vi "CRYAPI MSG PRO.vi"() -> ()   [LabVIEW 2013]
uses:
  CRYMain Sub Window Global.vi
  CRYProject/CRYProject Editor Global.vi
  CRYStepSetup/CRYStepSetup Global.vi
panel:
  in  "bStepRecovery":bool=TRUE
  in  "bOpenProjectFullPath":bool=TRUE
  in  "bStop":bool=TRUE
  in  "bMsg":bool=TRUE
  in  "nDData":i32
  in  "nSData":i32
  in  "sData":string="REMOTE_COMMAND"
  in  "nData":i32
  in  "pVI":refnum<vi>
  in  "sMsgCommand":string="REMOTE_COMMAND"
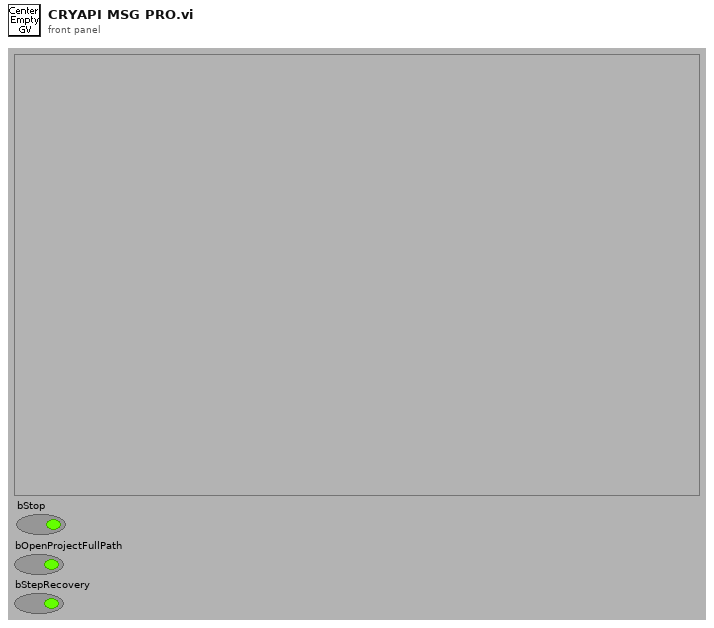
[diagram p1: front panel]
types:
  T1 = enum32{"Invalid", "Standard", "Closed", "Hidden", "Minimized", "Maximized"}
  T2 = typedef "LVRectTypeDef.ctl" = cluster{"Left":i16, "Top":i16, "Right":i16, "Bottom":i16}
  T3 = cluster{"nType":i32, "nParent":i32, "pVIW":refnum<vi>, "pSPW":refnum<vi>, "nTypeF":i32, "pVIF":refnum<vi>, "pSPF":refnum<vi>, "nIDSpliter":i32, "nProperty":i32, "Bound":T2, "nID":i32, "nData":i32, "sData":string, "pWVI":refnum<vi>, "sTitle":string, "cPages":cluster{"nPage":i32, "sTitle":string, "sIcon":string, "pVI":refnum<vi>, "nID":i32}[], "pTab":refnum<vi>, "nIDPages":i32[], "pSPT":refnum<vi>, "sTemp":string, "nDockID":i32, "nDockLR":i32, "sIcon":string}
  T4 = cluster{"EventName":string, "Arg1":string, "Numeric":u16, "Numeric 2":u16, "AddSteps ":refnum<vi>, "Arg1 2":string, "Arg1 3":string, "Boolean":bool}
  T5 = cluster{"sStepName":string, "nStepVINo":i32, "nStepVINoDisplay":i32}
  T6 = typedef "CRYTS.ctl" = cluster{"No.TS":u16, "TS File Path":path, "TS Name":string, "EditStepName":string, "Steps":T7[], "New State":bool, "Change State":bool, "Flattened CurveLib Data":string, "Document Data":string, "EditStepNo":u16, "Operator Start File":string, "Sequence Type":string, "Sequence Language":string}
  T7 = typedef "CRYStep.ctl" = cluster{"No.VI":i32, "Category":string, "StepName":string, "Seq setup flattened":string, "Comment":string, "Steps config.":bool[], "Jump config":i32[], "Start":dbl, "Increment":dbl, "Name":string, "Unit":string, "Y data":u16, "Y prefix":string, "Y dB ref":dbl, "Y unit":string, "Repeat State Array":cluster{"Start":dbl, "Increment":dbl, "Count":i32, "Num":i32}[]}
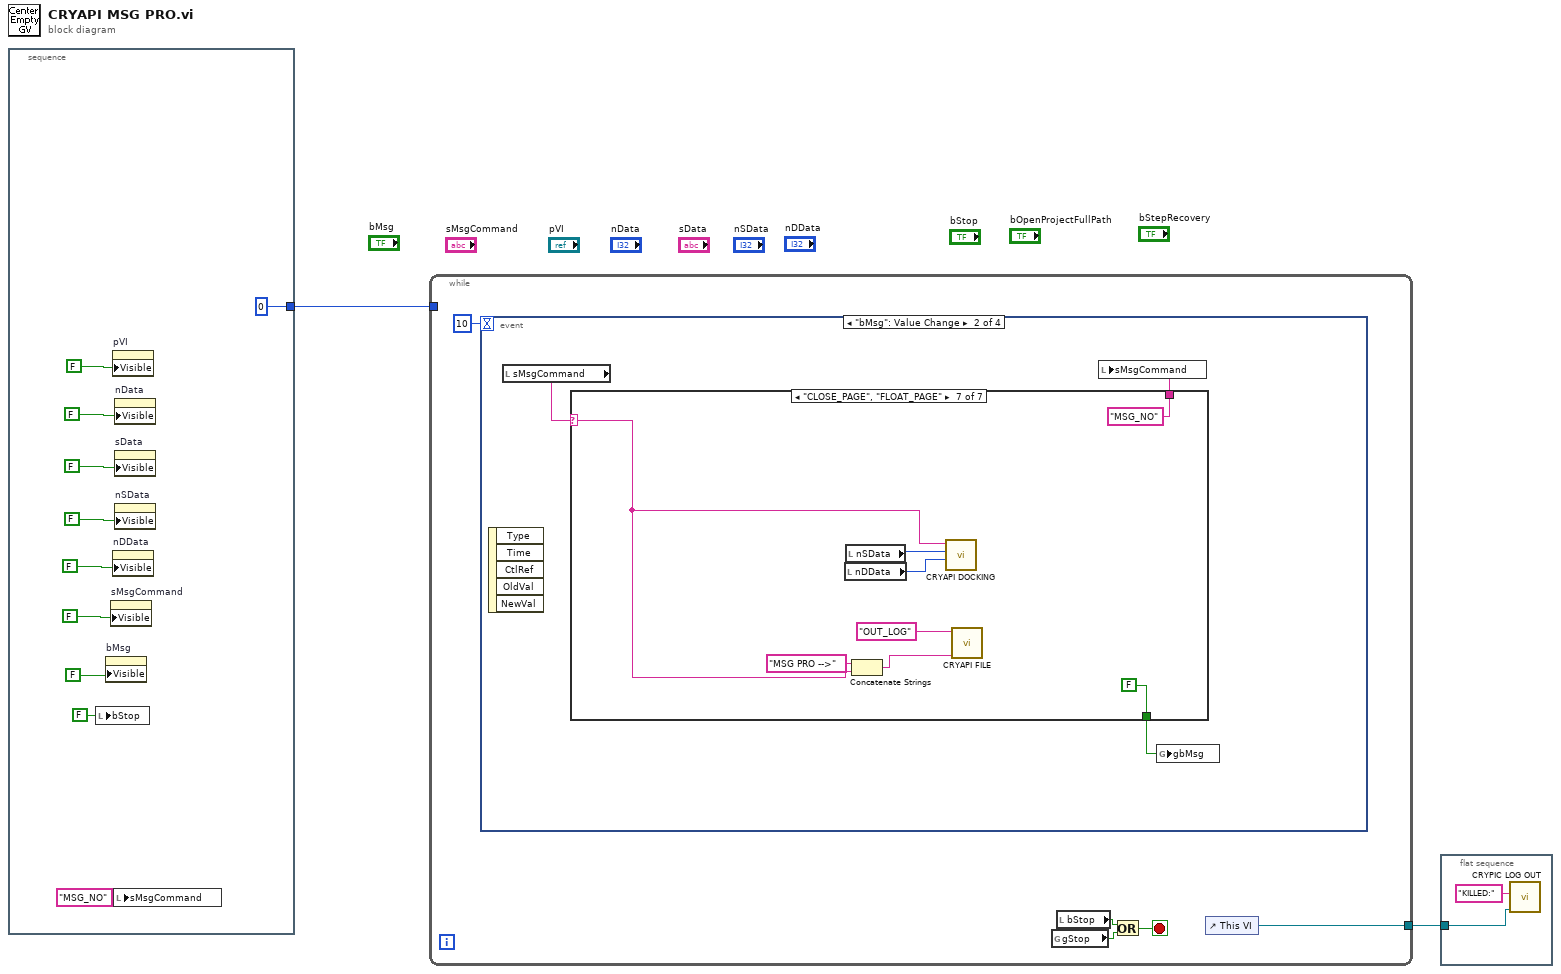
[diagram p0: block diagram]
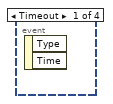
[diagram p2: hidden frame]
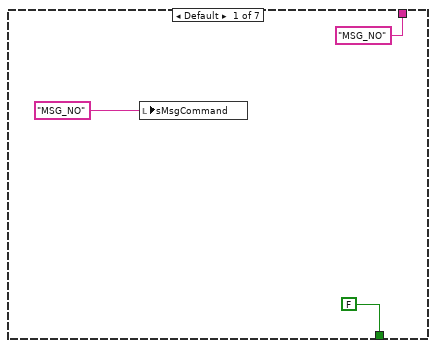
[diagram p3: hidden frame]
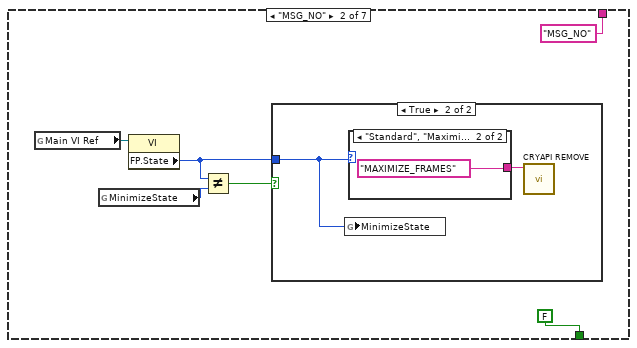
[diagram p4: hidden frame]
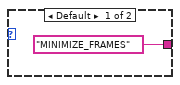
[diagram p6: hidden frame]
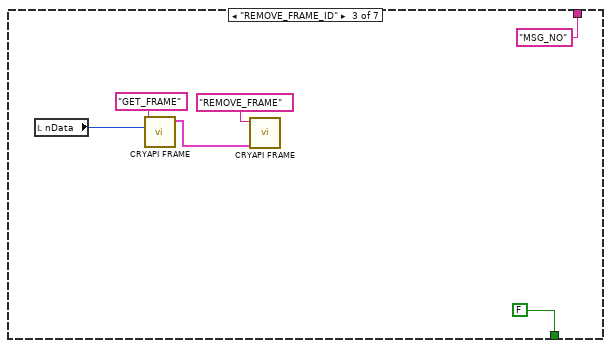
[diagram p7: hidden frame]
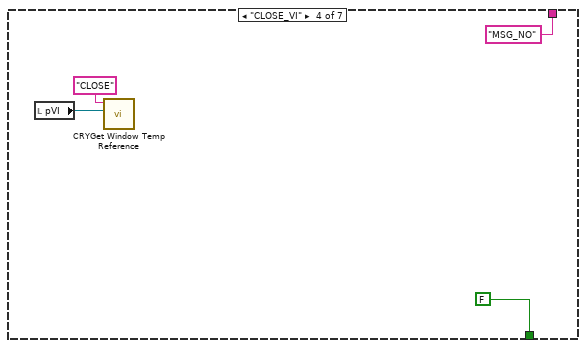
[diagram p8: hidden frame]
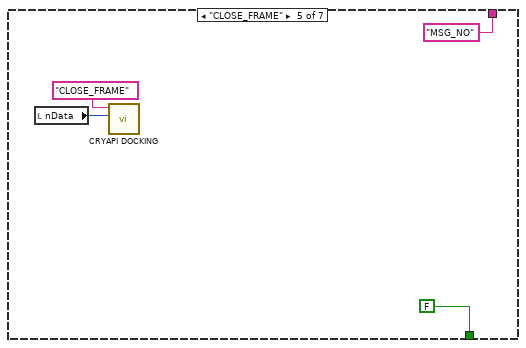
[diagram p9: hidden frame]
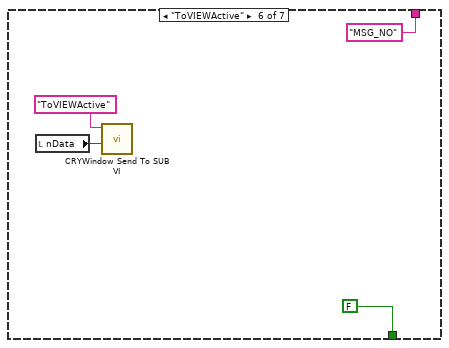
[diagram p10: hidden frame]
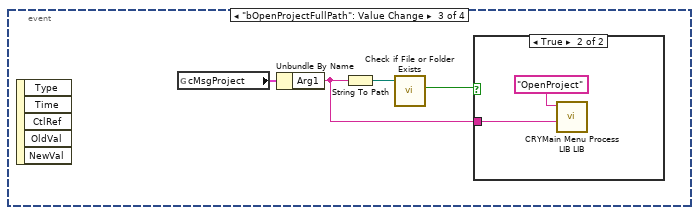
[diagram p11: hidden frame]
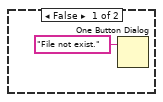
[diagram p12: hidden frame]
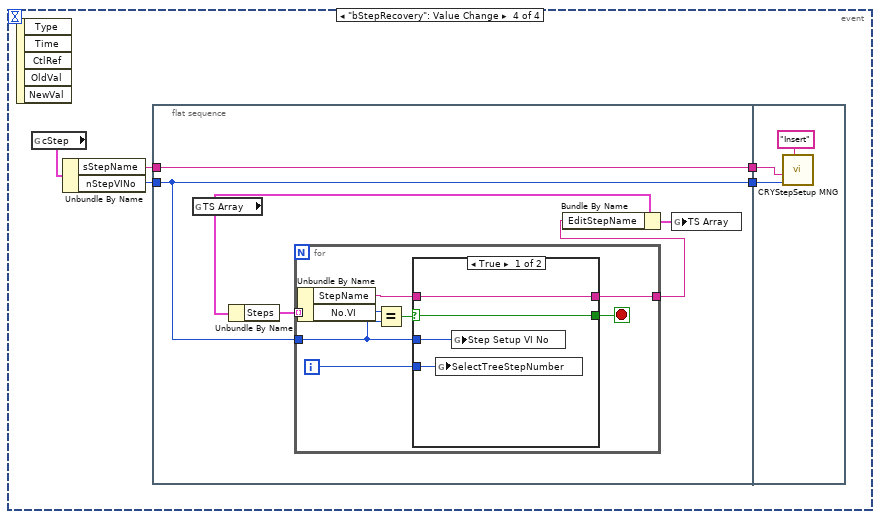
[diagram p13: hidden frame]
diagram:
  n1 = stacked-sequence {
    tunnel: [0] -> w2
    frame #0 {
      n2 = local write "bStop"(FALSE ("bStop")) -> ()
      n3 = property on="bMsg" class="Bool (strict)"("Visible"=FALSE) -> ()  [unwired: 2 in, 2 out]
      n4 = property on="sMsgCommand" class="Str"("Visible"=FALSE) -> ()  [unwired: 2 in, 2 out]
      n5 = property on="pVI" class="VIRef (strict)"("Visible"=FALSE) -> ()  [unwired: 2 in, 2 out]
      n6 = property on="nDData" class="DigNum (strict)"("Visible"=FALSE) -> ()  [unwired: 2 in, 2 out]
      n7 = local write "sMsgCommand"("MSG_NO" ("sAction")) -> ()
      n8 = property on="nData" class="DigNum (strict)"("Visible"=FALSE) -> ()  [unwired: 2 in, 2 out]
      n9 = property on="sData" class="Str"("Visible"=FALSE) -> ()  [unwired: 2 in, 2 out]
      n10 = property on="nSData" class="DigNum (strict)"("Visible"=FALSE) -> ()  [unwired: 2 in, 2 out]
    }
  }
  n11 = while {
    tunnel: w2 -> [_]
    tunnel: [w17] -> w1
    stop <- w16 stop-if-true
    n12 = event shown="[1] \"bMsg\": Value Change" {
      selector: _ -> [_ _ _ _]
      dyn-events: _ -> [_ _ _ _]
      timeout: 10 -> [_ _ _ _]
      event Timeout {
        n13 = event-data() -> ()  [unwired: 3 out]
      }
      event "bMsg": Value Change {
        n14 = event-data() -> ()  [unwired: 6 out]
        n15 = local read "sMsgCommand"() -> (w19:string)
        n16 = case shown="\"CLOSE_PAGE\", \"FLOAT_PAGE\"" w19 {
          selector: w19 -> [_ _ _ _ _ _ w52]
          tunnel: ["MSG_NO" ("sAction") "MSG_NO" ("sAction") "MSG_NO" ("sAction") "MSG_NO" ("sAction") "MSG_NO" ("sAction") "MSG_NO" ("sAction") "MSG_NO" ("sAction")] -> w18
          tunnel: [FALSE ("gbMsg") FALSE ("gbMsg") FALSE ("gbMsg") FALSE ("gbMsg") FALSE ("gbMsg") FALSE ("gbMsg") FALSE ("gbMsg")] -> w20
          frame Default {
            n17 = local write "sMsgCommand"("MSG_NO" ("sAction")) -> ()
          }
          frame "MSG_NO" {
            n18 = global read "CRYMain Sub Window Global.vi" "Main VI Ref"() -> (w25:refnum<vi>)
            n19 = global read "CRYMain Sub Window Global.vi" "MinimizeState"() -> (w28:T1)
            n20 = property class="VI"(reference=w25) -> ("FP.State"=w26:T1)  [unwired: 1 in, 2 out]
            n21 = Not Equal?(x=w26, y=w28) -> (x != y?=w27:bool)
            n22 = case shown="True" w27 {
              tunnel: w26 -> [_ w30]
              frame False {
              }
              frame True {
                n23 = global write "CRYMain Sub Window Global.vi" "MinimizeState"(w30) -> ()
                n24 = case shown="\"Standard\", \"Maximized\"" w30 {
                  tunnel: ["MINIMIZE_FRAMES" ("sAction") "MAXIMIZE_FRAMES" ("sAction")] -> w31
                  frame Default {
                  }
                  frame "Standard", "Maximized" {
                  }
                }
                n25 = call "CRYAPI REMOVE.vi"("sAction"=w31) -> ()  [unwired: 4 in, 7 out]
              }
            }
          }
          frame "REMOVE_FRAME_ID" {
            n26 = local read "nData"() -> (w36:i32)
            n27 = call "CRYAPI FRAME.vi"("nData"=w36, "sAction"="GET_FRAME") -> ("tFrame_Out"=w37:T3)  [unwired: 4 in, 5 out]
            n28 = call "CRYAPI FRAME.vi"("tFrame"=w37, "sAction"="REMOVE_FRAME") -> ()  [unwired: 4 in, 6 out]
          }
          frame "CLOSE_VI" {
            n29 = local read "pVI"() -> (w42:refnum<vi>)
            n30 = call "CRYGet Window Temp Reference.vi"("pVIRef_In"=w42, "sAction"="CLOSE") -> ()  [unwired: 2 in, 8 out]
          }
          frame "CLOSE_FRAME" {
            n31 = local read "nData"() -> (w47:i32)
            n32 = call "CRYAPI DOCKING.vi"("nSWinID"=w47, "sAction"="CLOSE_FRAME") -> ()  [unwired: 2 in, 8 out]
          }
          frame "ToVIEWActive" {
            n33 = local read "nData"() -> (w48:i32)
            n34 = call "CRYWindow Send To SUB VI.vi"("nData"=w48, "sAction"="ToVIEWActive") -> ()  [unwired: 9 in, 1 out]
          }
          frame "CLOSE_PAGE", "FLOAT_PAGE" {
            n35 = local read "nDData"() -> (w58:i32)
            n36 = local read "nSData"() -> (w59:i32)
            n37 = Concatenate Strings("MSG PRO -->" ("string"), w52) -> (w54:string)
            n38 = call "CRYAPI DOCKING.vi"("nDWinID"=w58, "nSWinID"=w59, "sAction"=w52) -> ()  [unwired: 2 in, 7 out]
            n39 = call "CRYAPI FILE.vi"("sData"=w54, "sAction"="OUT_LOG") -> ()  [unwired: 8 in, 2 out]
          }
        }
        n40 = local write "sMsgCommand"(w18) -> ()
        n41 = global write "CRYMain Sub Window Global.vi" "gbMsg"(w20) -> ()
      }
      event "bOpenProjectFullPath": Value Change {
        n42 = event-data() -> ()  [unwired: 6 out]
        n43 = global read "CRYProject Editor Global.vi" "cMsgProject"() -> (w63:T4)
        n44 = Unbundle By Name(w63) -> ("Arg1"=w60:string)
        n45 = String To Path(string=w60) -> (path=w62:path)
        n46 = call <vilib>:"Check if File or Folder Exists.vi"("path"=w62) -> ("file or folder exists?"=w61:bool)  [unwired: 8 in, 2 out]
        n47 = case shown="True" w61 {
          tunnel: w60 -> [_ w65]
          frame False {
            n48 = One Button Dialog(message="File not exist.") -> ()  [unwired: 1 in, 1 out]
          }
          frame True {
            n49 = call "CRYMain Menu Process LIB LIB.vi"("sOption"=w65, "sAction"="OpenProject") -> ()  [unwired: 9 in, 1 out]
          }
        }
      }
      event "bStepRecovery": Value Change {
        n50 = event-data() -> ()  [unwired: 6 out]
        n51 = global read "CRYStepSetup Global.vi" "cStep"() -> (w71:T5)
        n52 = Unbundle By Name(w71) -> ("sStepName"=w70:string, "nStepVINo"=w69:i32)
        n53 = flat-sequence {
          tunnel: w69 -> [w76]
          tunnel: w70 -> [w74]
          tunnel: [w74] -> w68
          tunnel: [w76] -> w67
          tunnel: w67 -> [w92]
          tunnel: w68 -> [w93]
          frame #0 {
            n54 = global read "CRYProject Editor Global.vi" "TS Array"() -> (w75:T6)
            n55 = Unbundle By Name(w75) -> ("Steps"=w77:T7[])
            n56 = for {
              tunnel: w77 -> [w85] mode=indexing
              tunnel: w76 -> [w81]
              tunnel: [w78] -> w72
              i -> [w80]
              stop <- w82 stop-if-true
              n57 = Unbundle By Name(w85) -> ("StepName"=w79:string, "No.VI"=w84:i32)
              n58 = Equal?(x=w84, y=w81) -> (x = y?=w83:bool)
              n59 = case shown="True" w83 {
                selector: w83 -> [w89 w91]
                tunnel: [w89 w91] -> w82
                tunnel: w81 -> [w88 _]
                tunnel: w80 -> [w87 _]
                tunnel: w79 -> [w86 w90]
                tunnel: [w86 w90] -> w78
                frame True {
                  n60 = global write "CRYProject Editor Global.vi" "SelectTreeStepNumber"(w87) -> ()
                  n61 = global write "CRYProject Editor Global.vi" "Step Setup VI No"(w88) -> ()
                }
                frame False {
                }
              }
            }
            n62 = Bundle By Name(cluster=w75, "EditStepName"=w72) -> (w73:T6)
            n63 = global write "CRYProject Editor Global.vi" "TS Array"(w73) -> ()
          }
          frame #1 {
            n64 = call "CRYStepSetup MNG.vi"("sAction"="Insert" ("sData"), "nData"=w92, "sStepName"=w93) -> ()  [unwired: 7 in, 2 out]
          }
        }
      }
    }
    n65 = global read "CRYMain Sub Window Global.vi" "gStop"() -> (w14:bool)
    n66 = local read "bStop"() -> (w15:bool)
    n67 = Or(x=w15, y=w14) -> (x .or. y?=w16:bool)
    n68 = control-ref of="This VI"() -> (w17:refnum<vi>)
  }
  n69 = flat-sequence {
    tunnel: w1 -> [w95]
    frame #0 {
      n70 = call "CRYPIC LOG OUT.vi"("pVIRef"=w95, "sData"="KILLED:") -> ()  [unwired: 10 in]
    }
  }
